vi "rspvtd_New Pumps Data.vi"(8 "error in":errorcluster, 11 "Data in":variant) -> (0 "error out":errorcluster, 3 "Data out":T1={"Насос"={"Давление заданное"=0.3, "Давление MAX заданное"=100.0, "Давление в насосе"=0.0, "Давление в системе"=99.99, "Расход заданый"=0.0, "Расход текущий"=0.0, "Объём заданный"=0.0, "Объём текущий"=0.0, "Позиция насоса %"=0.0, "Ток двигателя"=0.0, "controlMsg"="", "Клапан k_sys"=FALSE, "Клапан k_res"=FALSE, "Клапан k_air"=FALSE, "Вверх"=FALSE, "Домой"=FALSE, "Вниз"=FALSE, "Старт расход"=FALSE, "Старт давление"=FALSE, "Сброс объёма"=FALSE, "Сброс давления Рсис"=FALSE, "Сброс давления Рнас"=FALSE, "Bits"={"plc_control"=FALSE, "lag_control"=FALSE, "mstop_control"=FALSE, "st_home"=FALSE, "error"=FALSE, "mstart"=FALSE, "pair"=FALSE, "startQ"=FALSE, "startP"=FALSE, "volume_Stop"=FALSE}}, "Насос 2"={"Давление заданное"=0.3, "Давление MAX заданное"=100.0, "Давление в насосе"=0.0, "Давление в системе"=99.99, "Расход заданый"=0.0, "Расход текущий"=0.0, "Объём заданный"=0.0, "Объём текущий"=0.0, "Позиция насоса %"=0.0, "Ток двигателя"=0.0, "controlMsg"="", "Клапан k_sys"=FALSE, "Клапан k_res"=FALSE, "Клапан k_air"=FALSE, "Вверх"=FALSE, "Домой"=FALSE, "Вниз"=FALSE, "Старт расход"=FALSE, "Старт давление"=FALSE, "Сброс объёма"=FALSE, "Сброс давления Рсис"=FALSE, "Сброс давления Рнас"=FALSE, "Bits"={"plc_control"=FALSE, "lag_control"=FALSE, "mstop_control"=FALSE, "st_home"=FALSE, "error"=FALSE, "mstart"=FALSE, "pair"=FALSE, "startQ"=FALSE, "startP"=FALSE, "volume_Stop"=FALSE}}, "Насосная система"={"Давление заданное"=0.3, "Давление в системе"=99.99, "Расход заданый"=0.0, "Расход текущий"=0.0, "Объём заданный"=0.0, "Объём текущий"=0.0, "Старт давление"=FALSE, "Старт расход"=FALSE, "Сброс объёма"=FALSE, "plc_control"=FALSE, "lag_control"=FALSE, "mstop_control"=FALSE, "Давление"={"АЦП CH 0"=0.0, "АЦП CH 1"=0.0, "АЦП CH 2"=0.0, "АЦП CH 3"=0.0, "АЦП CH 4"=0.0, "АЦП CH 5"=0.0, "АЦП CH 6"=0.0, "АЦП CH 7"=0.0}, "Modbus"={"Массив чтения"=[], "Массив записи"=[]}}} {"Насосная система"."Давление"."АЦП CH 7" format="%.3f"; "Насосная система"."Давление"."АЦП CH 6" format="%.3f"; "Насосная система"."Давление"."АЦП CH 5" format="%.3f"; "Насосная система"."Давление"."АЦП CH 4" format="%.3f"; "Насосная система"."Давление"."АЦП CH 3" format="%.3f"; "Насосная система"."Давление"."АЦП CH 2" format="%.3f"; "Насосная система"."Давление"."АЦП CH 1" format="%.3f"; "Насосная система"."Давление"."АЦП CH 0" format="%.3f"; "Насосная система"."Объём текущий" min=0.0 max=9999.0 step=0.0001 format="%#_4f"; "Насосная система"."Объём заданный" min=0.0 max=9999.0 step=0.0001 format="%#_5f"; "Насосная система"."Расход текущий" format="%#_4f"; "Насосная система"."Расход заданый" min=-150.0 max=150.0 step=0.0001 format="%#_5f"; "Насосная система"."Давление в системе" format="%.2f"; "Насосная система"."Давление заданное" min=0.3 max=100.0 step=0.01 format="%#_5f"; "Насос 2"."Ток двигателя" format="%#_5f"; "Насос 2"."Расход текущий" format="%#_4f"; "Насос 2"."Давление в системе" format="%.2f"; "Насос 2"."Объём текущий" min=0.0 max=9999.0 step=0.0001 format="%#_4f"; "Насос 2"."Объём заданный" min=0.0 max=9999.0 step=0.0001 format="%#_5f"; "Насос 2"."Давление MAX заданное" min=0.0 max=100.0 step=0.01 format="%#_5f"; "Насос 2"."Давление заданное" min=0.3 max=100.0 step=0.01 format="%#_5f"; "Насос 2"."Расход заданый" min=-150.0 max=150.0 step=0.0001 format="%#_5f"; "Насос 2"."Давление в насосе" format="%.3f"; "Насос 2"."Позиция насоса %" scale=0.0..100.0 scale format="%.2f"; "Насос"."Ток двигателя" format="%#_5f"; "Насос"."Расход текущий" format="%#_4f"; "Насос"."Давление в системе" format="%.2f"; "Насос"."Объём текущий" min=0.0 max=9999.0 step=0.0001 format="%#_4f"; "Насос"."Объём заданный" min=0.0 max=9999.0 step=0.0001 format="%#_5f"; "Насос"."Давление MAX заданное" min=0.0 max=100.0 step=0.01 format="%#_5f"; "Насос"."Давление заданное" min=0.3 max=100.0 step=0.01 format="%#_5f"; "Насос"."Расход заданый" min=-150.0 max=150.0 step=0.0001 format="%#_5f"; "Насос"."Давление в насосе" format="%.3f"; "Насос"."Позиция насоса %" scale=0.0..100.0 scale format="%.2f"})   [LabVIEW 2023, in "pump_Lib.lvlib" / "Pumps Worker.lvclass"]
doc: "This VI converts variant data contained in the associated <b>Public API Response</b> message to its correct data type.\n---"
uses:
  Pumps Worker.lvclass
  rsp_New Pumps Data.ctl
  TypeDef/pump_Type_Pair_L.ctl
  TypeDef/pump_Type_Pair_R.ctl
  TypeDef/pair_Type.ctl
  pump_Lib.lvlib
panel:
  # "%"
  # "%"
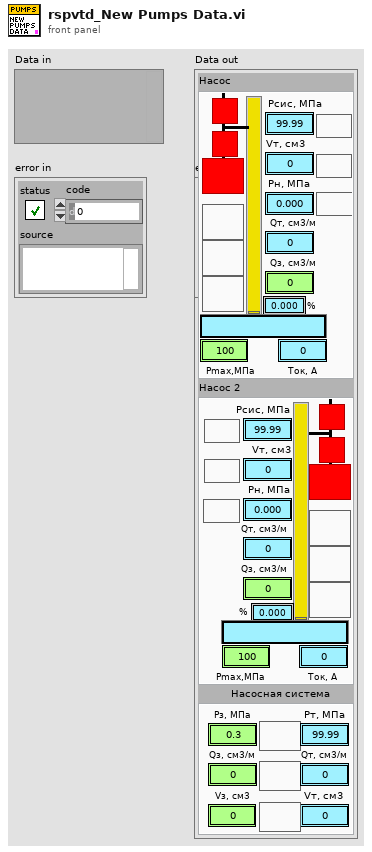
[diagram p1: front panel]
types:
  T1 = typedef "pump_Lib.lvlib/Pumps Worker.lvclass/rsp_New Pumps Data.ctl" = cluster{"Насос":T2, "Насос 2":T3, "Насосная система":T4}
  T2 = typedef "pump_Lib.lvlib/pump_Type_Pair_L.ctl" = cluster{"Давление заданное":dbl, "Давление MAX заданное":dbl, "Давление в насосе":dbl, "Давление в системе":dbl, "Расход заданый":dbl, "Расход текущий":dbl, "Объём заданный":dbl, "Объём текущий":dbl, "Позиция насоса %":dbl, "Ток двигателя":dbl, "controlMsg":string, "Клапан k_sys":bool, "Клапан k_res":bool, "Клапан k_air":bool, "Вверх":bool, "Домой":bool, "Вниз":bool, "Старт расход":bool, "Старт давление":bool, "Сброс объёма":bool, "Сброс давления Рсис":bool, "Сброс давления Рнас":bool, "Bits":cluster{"plc_control":bool, "lag_control":bool, "mstop_control":bool, "st_home":bool, "error":bool, "mstart":bool, "pair":bool, "startQ":bool, "startP":bool, "volume_Stop":bool}}
  T3 = typedef "pump_Lib.lvlib/pump_Type_Pair_R.ctl" = cluster{"Давление заданное":dbl, "Давление MAX заданное":dbl, "Давление в насосе":dbl, "Давление в системе":dbl, "Расход заданый":dbl, "Расход текущий":dbl, "Объём заданный":dbl, "Объём текущий":dbl, "Позиция насоса %":dbl, "Ток двигателя":dbl, "controlMsg":string, "Клапан k_sys":bool, "Клапан k_res":bool, "Клапан k_air":bool, "Вверх":bool, "Домой":bool, "Вниз":bool, "Старт расход":bool, "Старт давление":bool, "Сброс объёма":bool, "Сброс давления Рсис":bool, "Сброс давления Рнас":bool, "Bits":cluster{"plc_control":bool, "lag_control":bool, "mstop_control":bool, "st_home":bool, "error":bool, "mstart":bool, "pair":bool, "startQ":bool, "startP":bool, "volume_Stop":bool}}
  T4 = typedef "pump_Lib.lvlib/pair_Type.ctl" = cluster{"Давление заданное":dbl, "Давление в системе":dbl, "Расход заданый":dbl, "Расход текущий":dbl, "Объём заданный":dbl, "Объём текущий":dbl, "Старт давление":bool, "Старт расход":bool, "Сброс объёма":bool, "plc_control":bool, "lag_control":bool, "mstop_control":bool, "Давление":cluster{"АЦП CH 0":dbl, "АЦП CH 1":dbl, "АЦП CH 2":dbl, "АЦП CH 3":dbl, "АЦП CH 4":dbl, "АЦП CH 5":dbl, "АЦП CH 6":dbl, "АЦП CH 7":dbl}, "Modbus":cluster{"Массив чтения":u16[], "Массив записи":u16[]}}
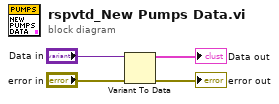
[diagram p0: block diagram]
diagram:
  n1 = Variant To Data(error in="error in", Variant="Data in") -> (data=→"Data out":T1, error out=→"error out":errorcluster)  [unwired: 1 in]
